vi "Get Return - Boolean.vi"(7 "Function Name":string, 8 "Error In":errorcluster, 11 "OPI Ref":refnum<data-value>) -> (0 "Error Out":errorcluster, 1 "Return Value":bool caption="Boolean", 3 "OPI Ref":refnum<data-value>)   [LabVIEW 2012, in "OPI.lvclass"]
doc: "Get return value from previously made function call, specified by Function Name. \n\nReturn a boolean."
uses:
  OPI.lvclass
  From Pythonic/From Pythonic - Boolean.vi
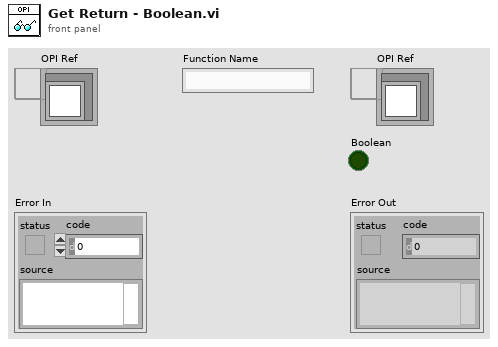
[diagram p1: front panel]
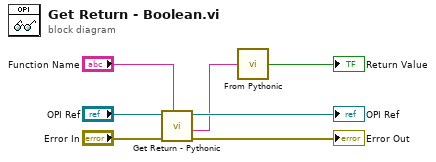
[diagram p0: block diagram]
diagram:
  n1 = call "Get Return - Pythonic.vi"("Function Name"="Function Name", "Error In"="Error In", "OPI Ref"="OPI Ref") -> ("Error Out"=→"Error Out":errorcluster, "Pythonic Return Value"=w2:string, "OPI Ref"=→"OPI Ref":refnum<data-value>)  [unwired: 6 in]
  n2 = call-poly "From Pythonic.vi"("Pythonic Value"=w2) -> ("Boolean"=→"Return Value":bool)  [unwired: 4 in]
